vi "find all occurences.vi"(3 "start index (0)":i32, 4 "element":dbl, 5 "1D array":dbl[](array[numeric])) -> (0 "number of occurances":i32, 2 "indexes":i32[](array[numeric]))   [LabVIEW 2009]
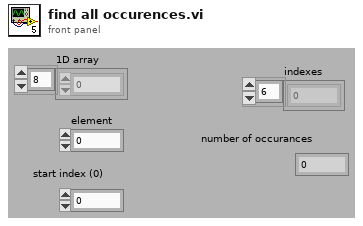
[diagram p1: front panel]
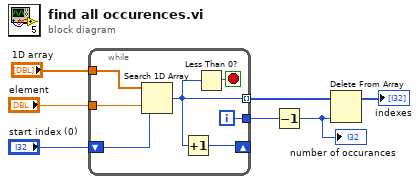
[diagram p0: block diagram]
diagram:
  n1 = while {
    tunnel: "1D array" -> [w12]
    tunnel: "element" -> [w13]
    tunnel: [w9] -> w4 mode=indexing
    shift-right: [w11] -> _
    shift-left: "start index (0)" -> [w14]
    tunnel: [w8] -> w1
    i -> [w8]
    stop <- w10 stop-if-true
    n2 = Search 1D Array(1D array=w12, element=w13, start index (0)=w14) -> (index of element=w9:i32)
    n3 = Increment(x=w9) -> (x+1=w11:i32)
    n4 = Less Than 0?(x=w9) -> (x < 0?=w10:bool)
  }
  n5 = Decrement(x=w1) -> (x-1=w2:i32)
  "number of occurances" <- w2
  n6 = Delete From Array(array=w4, index=w2) -> (array with subset deleted=→"indexes":i32[])  [unwired: 1 in, 1 out]
